vi "str_lineformat.vi"(6 "Format String":string[](array[string])=["000", "001", "002"], 8 "Timestamp":dbl, 10 "String Array":string[](array[string])) -> (2 "Formatted String":string)   [LabVIEW 2018]
doc: "Formats an array of strings into a single line string with tabs between each element of the array. Terminates the line with a line feed."
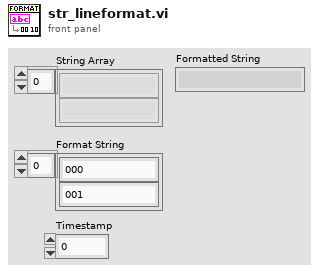
[diagram p1: front panel]
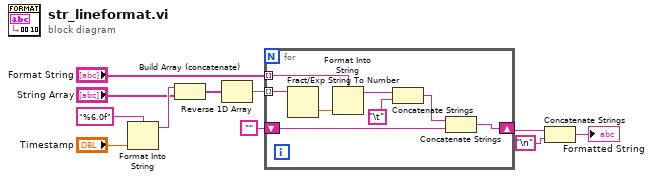
[diagram p0: block diagram]
diagram:
  n1 = Format Into String(format string="%6.0f", "Timestamp") -> (resulting string=w3:string)  [unwired: 2 in, 1 out]
  n2 = Build Array (concatenate)(w3, "String Array") -> (w4:string[])
  n3 = Reverse 1D Array(array=w4) -> (reversed array=w8:string[])
  n4 = for {
    shift-right: [w18] -> w10
    shift-left: "" -> [w17]
    tunnel: w8 -> [w15] mode=indexing
    tunnel: "Format String" -> [w12] mode=indexing
    n5 = Fract/Exp String To Number(string=w15) -> (number=w14:dbl)  [unwired: 3 in, 1 out]
    n6 = Format Into String(format string=w12, w14) -> (resulting string=w13:string)  [unwired: 2 in, 1 out]
    n7 = Concatenate Strings(w13, "\t") -> (w19:string)
    n8 = Concatenate Strings(w19, w17) -> (w18:string)
  }
  n9 = Concatenate Strings(w10, "\n") -> (→"Formatted String":string)
